vi "dfd_Utility I32 x I32.vi"(2 "y[I32]":i32=-5678, 3 "x [I32]":i32=-32767) -> (0 "x*y [Lo U32]":u32=59858, 1 "x*y [Hi I32]":i32=2838)   [LabVIEW 2017, in "NI_DigFilterLicensed.lvlib"]
uses:
  <vilib>/addons/Digital Filter Design/NI_DigFilterLicensed.lvlib
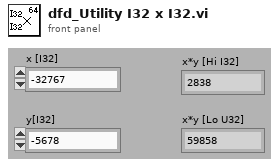
[diagram p1: front panel]
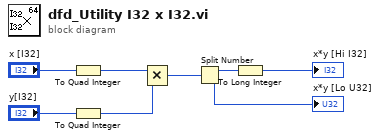
[diagram p0: block diagram]
diagram:
  n1 = To Quad Integer(1:"x [I32]") -> (0:w6:i64)
  n2 = To Quad Integer(1:"y[I32]") -> (0:w5:i64)
  n3 = Multiply(x=w6, y=w5) -> (x*y=w4:i64)
  n4 = Split Number(x=w4) -> (hi(x)=w3:u32, lo(x)=→"x*y [Lo U32]":u32)
  n5 = To Long Integer(number=w3) -> (32bit integer=→"x*y [Hi I32]":i32)
